vi "Start Command.vi"(8 "error in (no error)":errorcluster, 11 "ReceiveCommand in":refnum<class "Connect Command.lvclass">) -> (0 "error out":errorcluster, 3 "ReceiveCommand out":refnum<class "Connect Command.lvclass">)   [LabVIEW 2013, in "Receiver.lvlib" / "Receive Commands Using State Actors.lvlib" / "Connect Command.lvlib" / "Connect Command.lvclass"]
uses:
  Connect Command.lvclass
  Receiver Commands/Receiver Command.lvclass
  <vilib>/ActorFramework/Actor/Actor.lvclass
  Connect Command Messages/Go To Annoucing Msg/Go To Annoucing Msg.lvclass
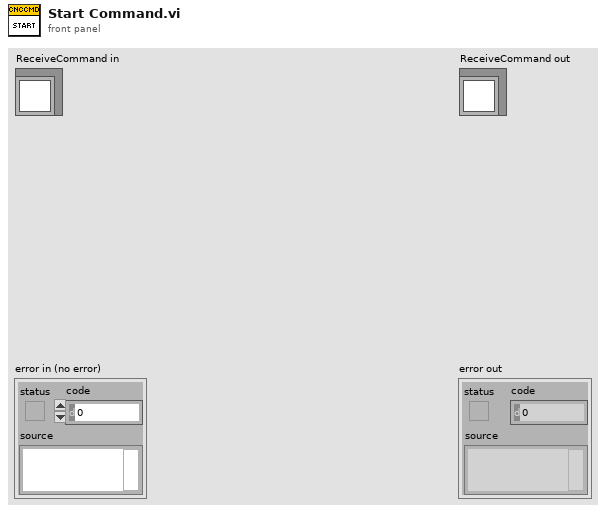
[diagram p1: front panel]
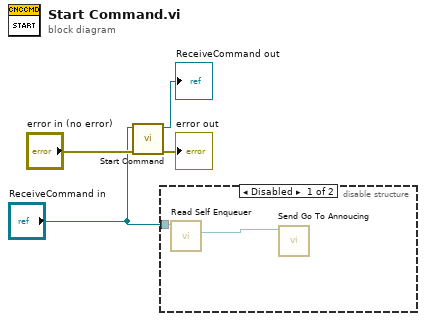
[diagram p0: block diagram]
diagram:
  n1 = call-parent "Start Command.vi"("error in (no error)"="error in (no error)", "Command in"="ReceiveCommand in") -> ("error out"=→"error out":errorcluster, "Command out"=→"ReceiveCommand out":refnum<class "Connect Command.lvclass">)  [unwired: 8 in]
  n2 = disable-structure shown="Disabled" {
    disable-tunnel: "ReceiveCommand in" -> [w6 _]
    frame Disabled {
      n3 = call <vilib>:"Read Self Enqueuer.vi"("Actor"=w6) -> ("Self Enqueuer"=w5:refnum<class "Message Enqueuer.lvclass">)  [unwired: 10 in]
      n4 = call "Send Go To Annoucing.vi"("Message Enqueuer"=w5) -> ()  [unwired: 9 in, 2 out]
    }
    frame Enabled {
    }
  }
